vi "filter.filter.add.vi"(11 "filter.data in":T1 {"memory.command"."order.slot.value"."Quantity" format="%016x"; "memory.command"."order.slot.value"."OrderId" format="%016x"; "memory.command"."ticker.slot.value"."Symbol" format="%016x"; "Scratch"."OrderId" format="%016x"}) -> (3 "filter.data out":T1 {"memory.command"."order.slot.value"."Quantity" format="%016x"; "memory.command"."order.slot.value"."OrderId" format="%016x"; "memory.command"."ticker.slot.value"."Symbol" format="%016x"; "Scratch"."OrderId" format="%016x"})   [LabVIEW 2022 SP3]
uses:
  filter.data.ctl
  filter.states.ctl
  filter.debug.ctl
  filter.debug.slot.ctl
  filter.data.scratch.ctl
  common/orderbook.command.ctl
  common/orderbook.command.type.ctl
  filter.memory.command.ctl
  ticker.slot.ctl
  order.slot.ctl
  filter.getstate.ctl
  filter.getstate.slot.ctl
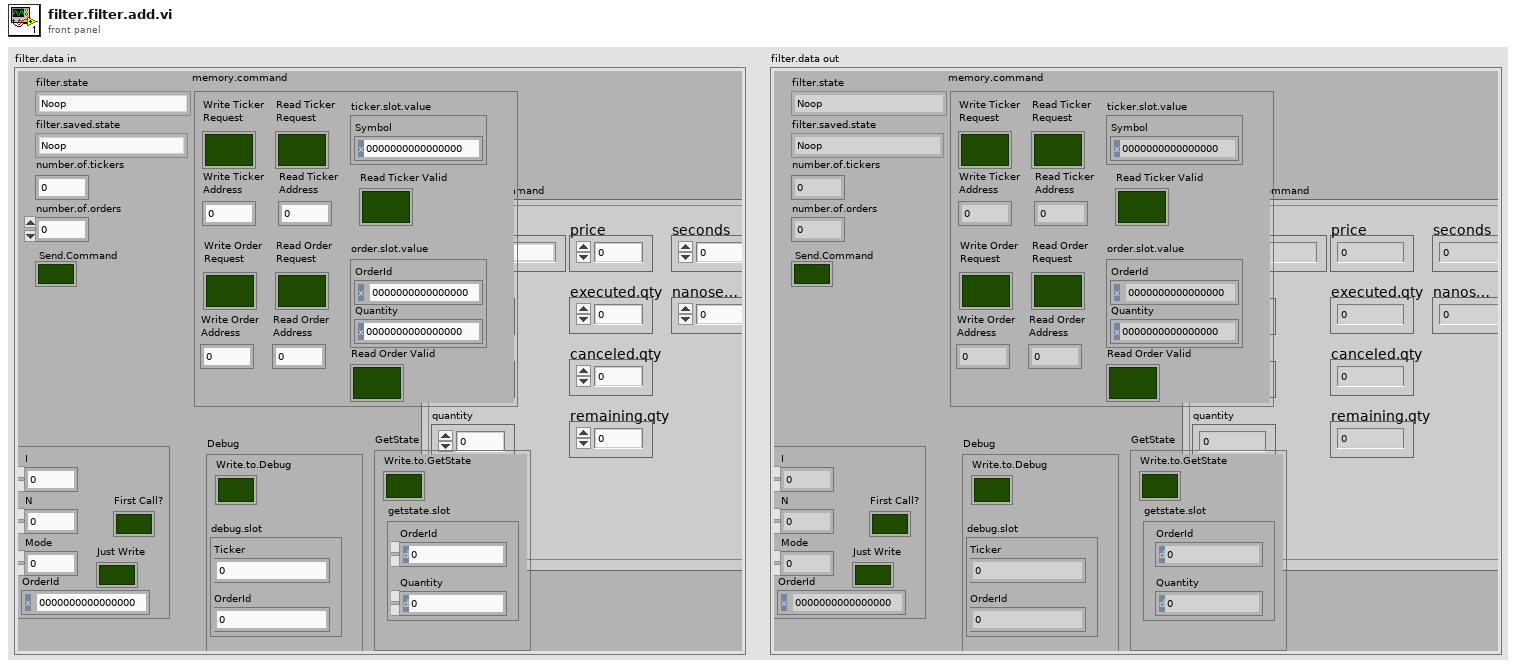
[diagram p1: front panel]
types:
  T1 = typedef "filter.data.ctl" = cluster{"filter.state":T2, "Debug":T3, "number.of.tickers":u32, "number.of.orders":u32, "filter.saved.state":T2, "Scratch":T5, "OrderBook.Command":T6, "Send.Command":bool, "memory.command":T8, "GetState":T11}
  T2 = typedef "filter.states.ctl" = enum16{"Noop", "Reset", "Debug", "Configuration", "Get.State", "Wait.for.Command", "Filter.Add", "Filter.Other", "Insert.Order", "Delete Order"}
  T3 = typedef "filter.debug.ctl" = cluster{"Write.to.Debug":bool, "debug.slot":T4}
  T4 = typedef "filter.debug.slot.ctl" = cluster{"Ticker":u64, "OrderId":u64}
  T5 = typedef "filter.data.scratch.ctl" = cluster{"I":u32, "N":u32, "Mode":u32, "OrderId":u64, "First Call?":bool, "Just Write":bool}
  T6 = typedef "orderbook.command.ctl" = cluster{"type":T7, "side":u8, "orderId ":u64, "quantity":u32, "symbol":u64, "price":u64, "executed.qty":u32, "canceled.qty":u32, "remaining.qty":u32, "seconds":u64, "nanoseconds":u64}
  T7 = typedef "orderbook.command.type.ctl" = enum8{"Time", "AddOrder", "OrderExecuted", "OrderExecutedAtPrice", "ReduceSize", "ModifyOrder", "DeleteOrder", "Get.State", "Get.All.Orders", "Get.Top"}
  T8 = typedef "filter.memory.command.ctl" = cluster{"ticker.slot.value":T9, "order.slot.value":T10, "Write Ticker\nAddress":u32, "Write Ticker\nRequest":bool, "Read Ticker\nRequest":bool, "Read Ticker\nAddress":u32, "Read Ticker Valid":bool, "Write Order\nAddress":u32, "Write Order\nRequest":bool, "Read Order\nRequest":bool, "Read Order\nAddress":u32, "Read Order Valid":bool}
  T9 = typedef "ticker.slot.ctl" = cluster{"Symbol":u64}
  T10 = typedef "order.slot.ctl" = cluster{"OrderId":u64, "Quantity":u64}
  T11 = typedef "filter.getstate.ctl" = cluster{"Write.to.GetState":bool, "getstate.slot":T12}
  T12 = typedef "filter.getstate.slot.ctl" = cluster{"OrderId":u64, "Quantity":u64}
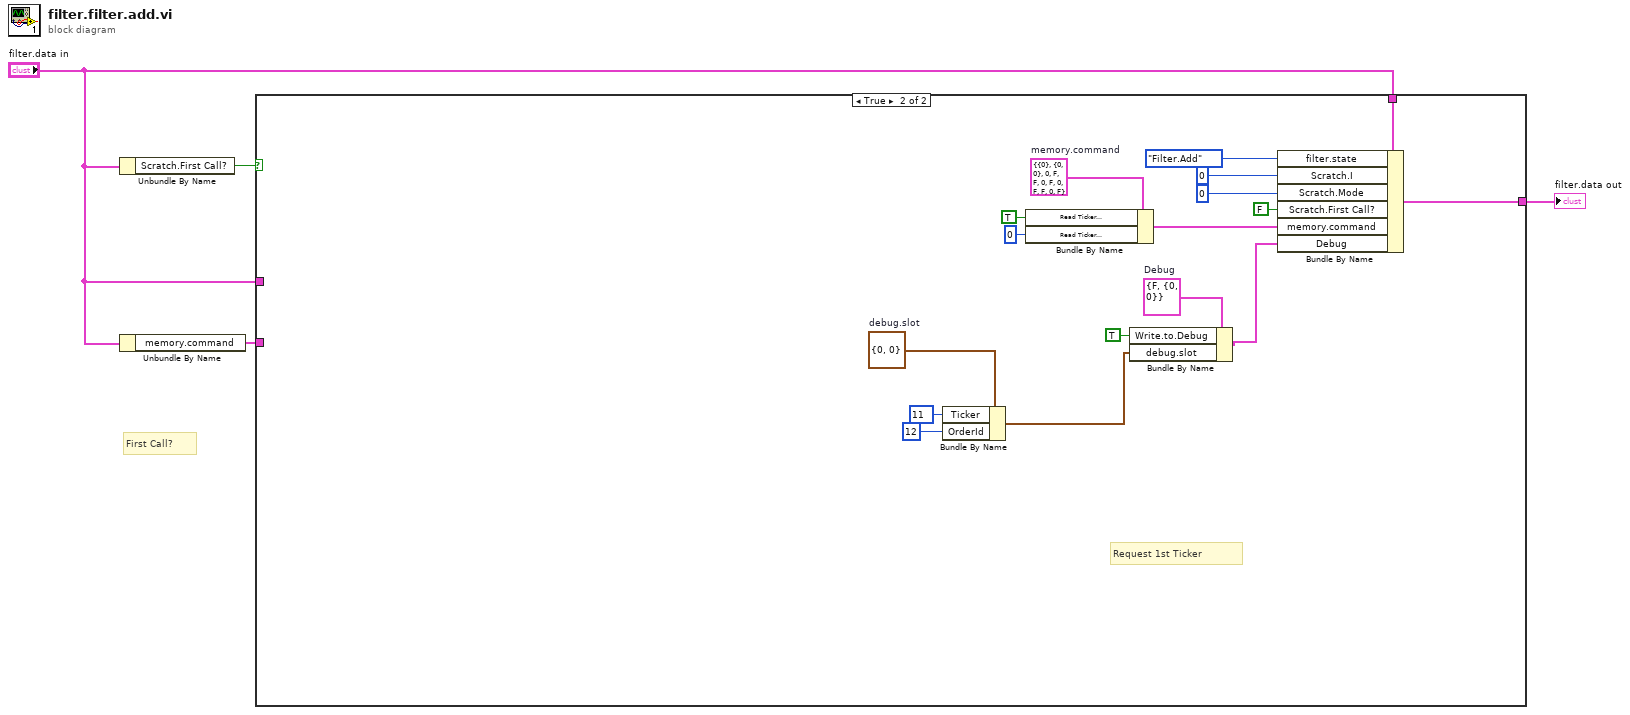
[diagram p0: block diagram]
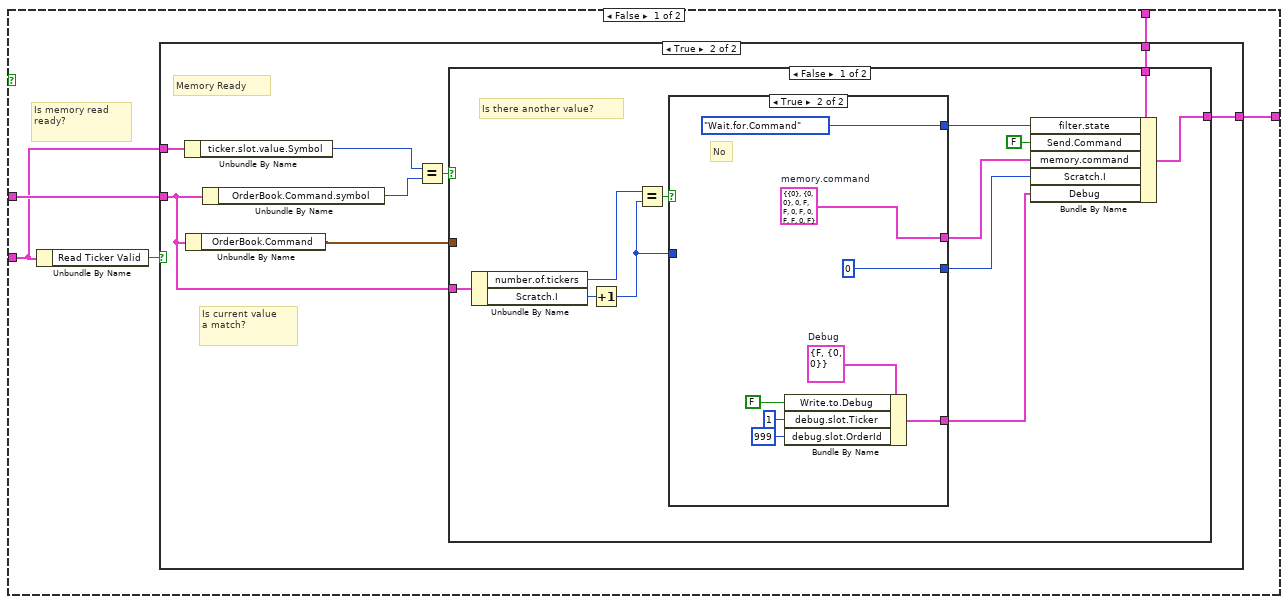
[diagram p2: hidden frame]
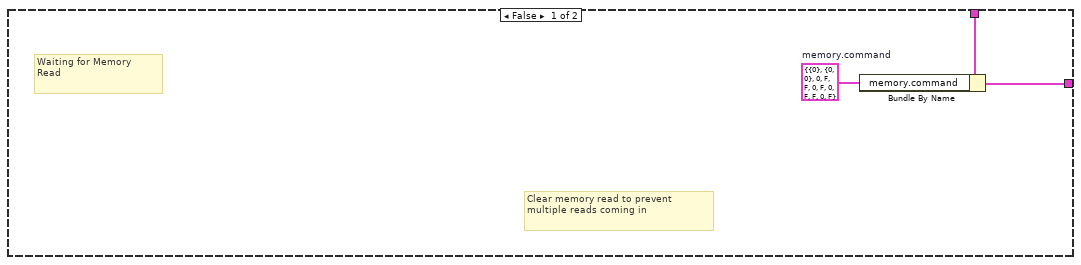
[diagram p3: hidden frame]
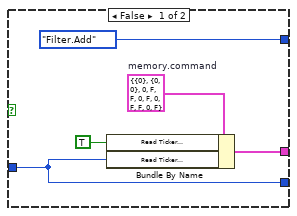
[diagram p4: hidden frame]
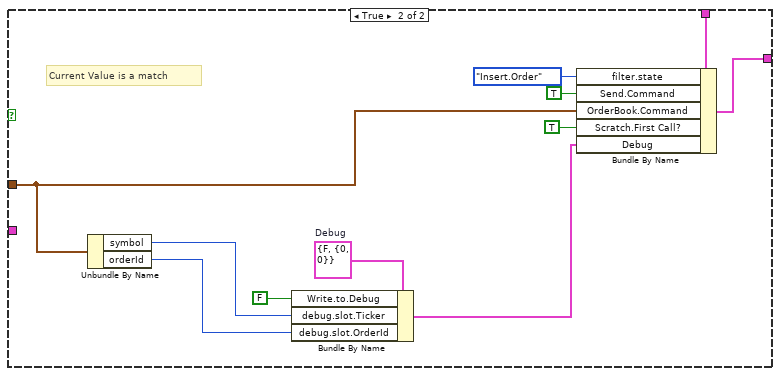
[diagram p5: hidden frame]
diagram:
  # "First Call?"
  n1 = Unbundle By Name("filter.data in") -> ("Scratch.First Call?"=w1:bool)
  n2 = Unbundle By Name("filter.data in") -> ("memory.command"=w3:T8)
  n3 = case shown="True" w1 {
    tunnel: "filter.data in" -> [w7 w73]
    tunnel: [w8 w71] -> w2
    tunnel: w3 -> [w5 _]
    tunnel: "filter.data in" -> [w6 _]
    frame False {
      # "Is memory read\nready?"
      n4 = Unbundle By Name(w5) -> ("Read Ticker Valid"=w9:bool)
      n5 = case shown="True" w9 {
        tunnel: [w10 w17] -> w8
        tunnel: w7 -> [w12 w18]
        tunnel: w6 -> [_ w15]
        tunnel: w5 -> [_ w20]
        frame False {
          w11 = T8 {"ticker.slot.value"={"Symbol"=0}, "order.slot.value"={"OrderId"=0, "Quantity"=0}, "Write Ticker\nAddress"=0, "Write Ticker\nRequest"=FALSE, "Read Ticker\nRequest"=FALSE, "Read Ticker\nAddress"=0, "Read Ticker Valid"=FALSE, "Write Order\nAddress"=0, "Write Order\nRequest"=FALSE, "Read Order\nRequest"=FALSE, "Read Order\nAddress"=0, "Read Order Valid"=FALSE}  # memory.command
          # "Clear memory read to prevent\nmultiple reads coming in"
          # "Waiting for Memory\nRead"
          n6 = Bundle By Name(cluster=w12, "memory.command"=w11) -> (w10:T1)
        }
        frame True {
          # "Is current value\na match?"
          # "Memory Ready"
          n7 = Unbundle By Name(w20) -> ("ticker.slot.value.Symbol"=w13:u64)
          n8 = Unbundle By Name(w15) -> ("OrderBook.Command"=w16:T6)
          n9 = Unbundle By Name(w15) -> ("OrderBook.Command.symbol"=w14:u64)
          n10 = Equal?(x=w13, y=w14) -> (x = y?=w19:bool)
          n11 = case shown="False" w19 {
            tunnel: w18 -> [w31 w56]
            tunnel: [w32 w54] -> w17
            tunnel: w16 -> [_ w48]
            tunnel: w15 -> [w30 _]
            frame False {
              # "Is there another value?"
              n12 = Unbundle By Name(w30) -> ("number.of.tickers"=w28:u32, "Scratch.I"=w29:u32)
              n13 = Increment(x=w29) -> (x+1=w25:u32)
              n14 = Equal?(x=w28, y=w25) -> (x = y?=w26:bool)
              n15 = case shown="True" w26 {
                tunnel: [w35 w44] -> w27
                tunnel: w25 -> [w33 _]
                tunnel: [filter.states."Filter.Add" ("filter.state") filter.states."Wait.for.Command" ("filter.state")] -> w24
                tunnel: [w33 u32 0] -> w22
                tunnel: [_ w40] -> w21
                frame False {
                  w37 = T8 {"ticker.slot.value"={"Symbol"=0}, "order.slot.value"={"OrderId"=0, "Quantity"=0}, "Write Ticker\nAddress"=0, "Write Ticker\nRequest"=FALSE, "Read Ticker\nRequest"=FALSE, "Read Ticker\nAddress"=0, "Read Ticker Valid"=FALSE, "Write Order\nAddress"=0, "Write Order\nRequest"=FALSE, "Read Order\nRequest"=FALSE, "Read Order\nAddress"=0, "Read Order Valid"=FALSE}  # memory.command
                  n16 = Bundle By Name(cluster=w37, "Read Ticker\nRequest"=TRUE ("ticker.slot"), "Read Ticker\nAddress"=w33) -> (w35:T8)
                }
                frame True {
                  w42 = T3 {"Write.to.Debug"=FALSE, "debug.slot"={"Ticker"=0, "OrderId"=0}}  # Debug
                  w44 = T8 {"ticker.slot.value"={"Symbol"=0}, "order.slot.value"={"OrderId"=0, "Quantity"=0}, "Write Ticker\nAddress"=0, "Write Ticker\nRequest"=FALSE, "Read Ticker\nRequest"=FALSE, "Read Ticker\nAddress"=0, "Read Ticker Valid"=FALSE, "Write Order\nAddress"=0, "Write Order\nRequest"=FALSE, "Read Order\nRequest"=FALSE, "Read Order\nAddress"=0, "Read Order Valid"=FALSE}  # memory.command
                  # "No"
                  n17 = Bundle By Name(cluster=w42, "Write.to.Debug"=FALSE, "debug.slot.Ticker"=u64 1, "debug.slot.OrderId"=u64 999) -> (w40:T3)
                }
              }
              n18 = Bundle By Name(cluster=w31, "filter.state"=w24, "Send.Command"=FALSE, "memory.command"=w27, "Scratch.I"=w22, "Debug"=w21) -> (w32:T1)
            }
            frame True {
              w51 = T3 {"Write.to.Debug"=FALSE, "debug.slot"={"Ticker"=0, "OrderId"=0}}  # Debug
              # "Current Value is a match"
              n19 = Unbundle By Name(w48) -> ("symbol"=w46:u64, "orderId"=w47:u64)
              n20 = Bundle By Name(cluster=w51, "Write.to.Debug"=FALSE, "debug.slot.Ticker"=w46, "debug.slot.OrderId"=w47) -> (w49:T3)
              n21 = Bundle By Name(cluster=w56, "filter.state"=filter.states."Insert.Order", "Send.Command"=TRUE, "OrderBook.Command"=w48, "Scratch.First Call?"=TRUE, "Debug"=w49) -> (w54:T1)
            }
          }
        }
      }
    }
    frame True {
      w59 = T4 {"Ticker"=0, "OrderId"=0}  # debug.slot
      w63 = T3 {"Write.to.Debug"=FALSE, "debug.slot"={"Ticker"=0, "OrderId"=0}}  # Debug
      w70 = T8 {"ticker.slot.value"={"Symbol"=0}, "order.slot.value"={"OrderId"=0, "Quantity"=0}, "Write Ticker\nAddress"=0, "Write Ticker\nRequest"=FALSE, "Read Ticker\nRequest"=FALSE, "Read Ticker\nAddress"=0, "Read Ticker Valid"=FALSE, "Write Order\nAddress"=0, "Write Order\nRequest"=FALSE, "Read Order\nRequest"=FALSE, "Read Order\nAddress"=0, "Read Order Valid"=FALSE}  # memory.command
      # "Request 1st Ticker"
      n22 = Bundle By Name(cluster=w59, "Ticker"=u64 11, "OrderId"=u64 12) -> (w60:T4)
      n23 = Bundle By Name(cluster=w70, "Read Ticker\nRequest"=TRUE ("Read.Request"), "Read Ticker\nAddress"=u32 0 ("Address")) -> (w67:T8)
      n24 = Bundle By Name(cluster=w63, "Write.to.Debug"=TRUE, "debug.slot"=w60) -> (w61:T3)
      n25 = Bundle By Name(cluster=w73, "filter.state"=filter.states."Filter.Add", "Scratch.I"=u32 0, "Scratch.Mode"=u32 0, "Scratch.First Call?"=FALSE, "memory.command"=w67, "Debug"=w61) -> (w71:T1)
    }
  }
  "filter.data out" <- w2
